vi "maszyna stanowa 1.vi"(6 "Niewykonane eventy in":T1[](array[typedef]), 8 "Ile godzin":i32=1, 9 "Liczba klientów na godzinę":i32=100, 10 "Sklep in":T2={"kasy"=2, "wolne"=2, "zarobek"=0, "liczba klientów"=0, "czas w kolejce"=0}, 11 "queue in":refnum<queue>) -> (0 "Straceni klienci":i32, 1 "Niewykonane eventy out":T1[](array[typedef]), 2 "Sklep out":T2={"kasy"=2, "wolne"=2, "zarobek"=0, "liczba klientów"=0, "czas w kolejce"=0}, 3 "queue out":refnum<queue>)   [LabVIEW 2013]
uses:
  event.ctl
  sklep.ctl
panel:
  out "liczba klientów":i32
  out "zarobek":i32
  out "średni czas w kolejce":dbl
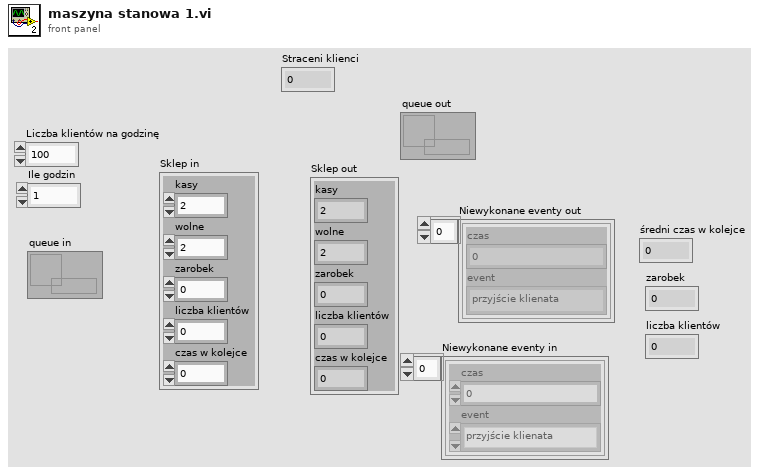
[diagram p1: front panel]
types:
  T1 = typedef "event.ctl" = cluster{"czas":u32, "event":enum16{"przyjście klienata", "zwolnienie kasy", "oczekiwanie na klienta", "nowy event"}}
  T2 = typedef "sklep.ctl" = cluster{"kasy":i32, "wolne":i32, "zarobek":i32, "liczba klientów":i32, "czas w kolejce":u64}
  T3 = enum16{"przyjście klienata", "zwolnienie kasy", "oczekiwanie na klienta", "nowy event"}
  T4 = cluster{dbl, "event":enum16{"przyjście klienata", "zwolnienie kasy", "oczekiwanie na klienta", "nowy event"}}
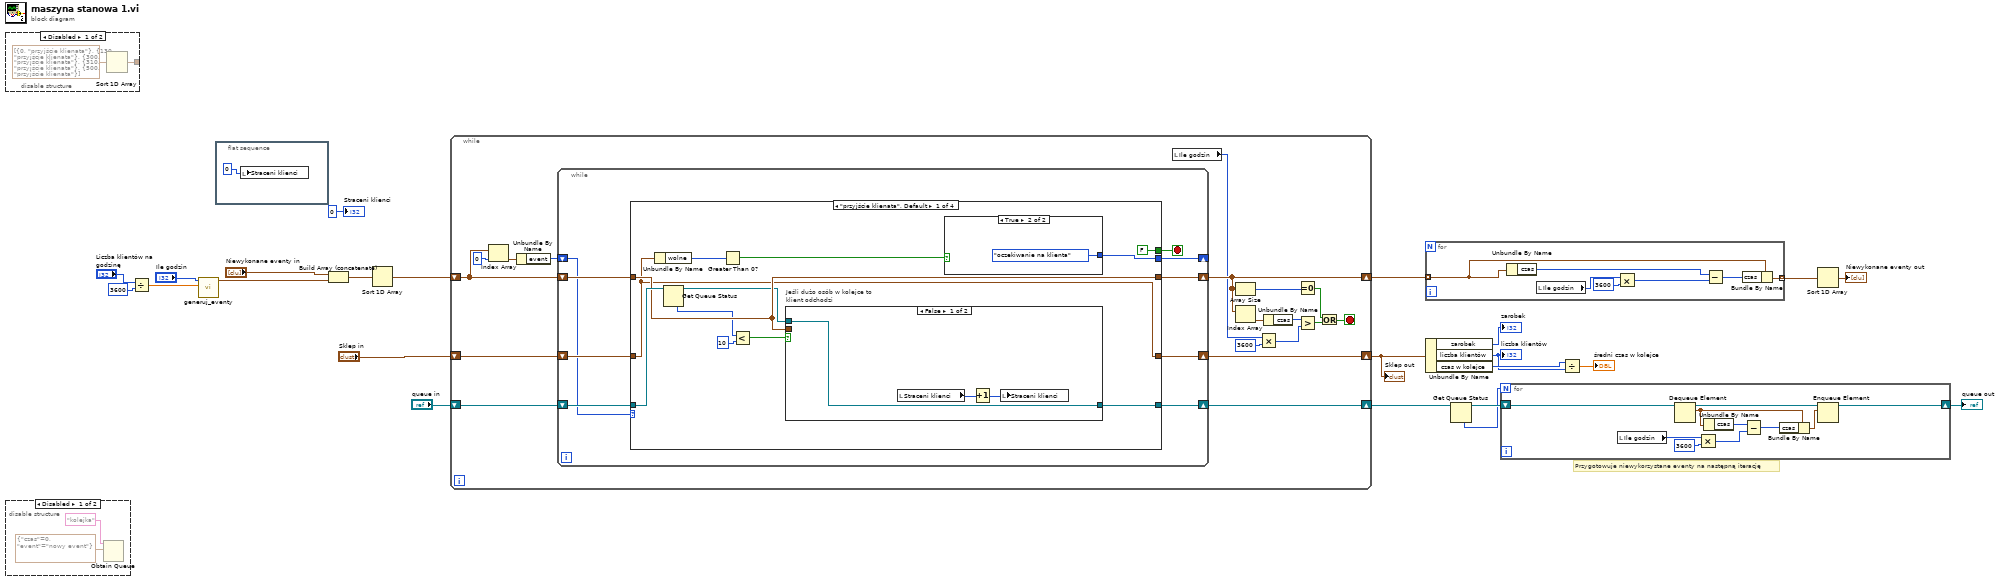
[diagram p0: block diagram]
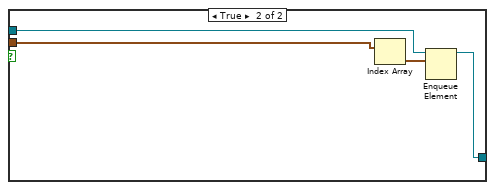
[diagram p4: hidden frame]
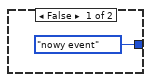
[diagram p5: hidden frame]
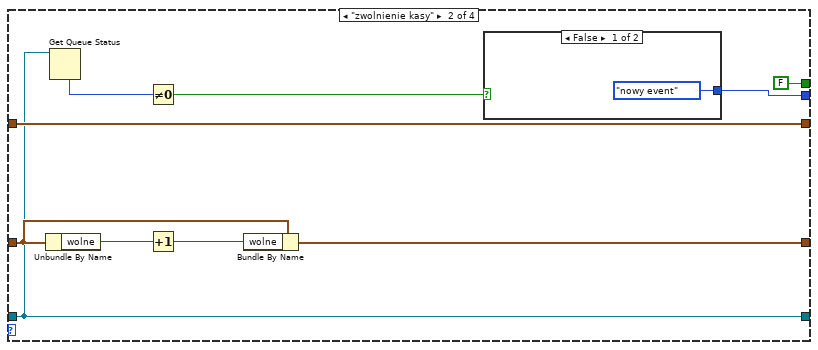
[diagram p6: hidden frame]
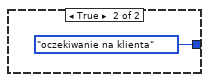
[diagram p7: hidden frame]
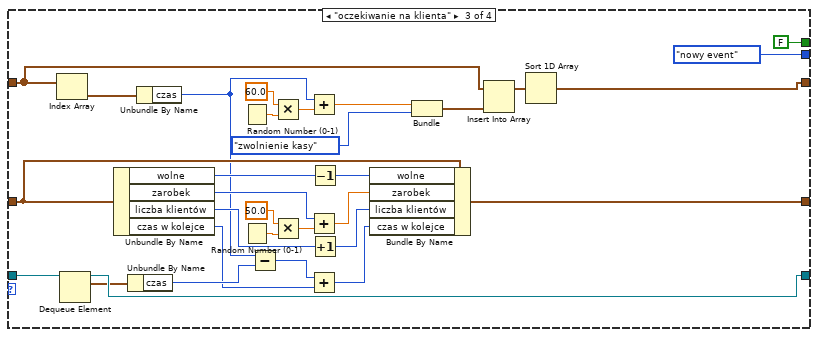
[diagram p8: hidden frame]
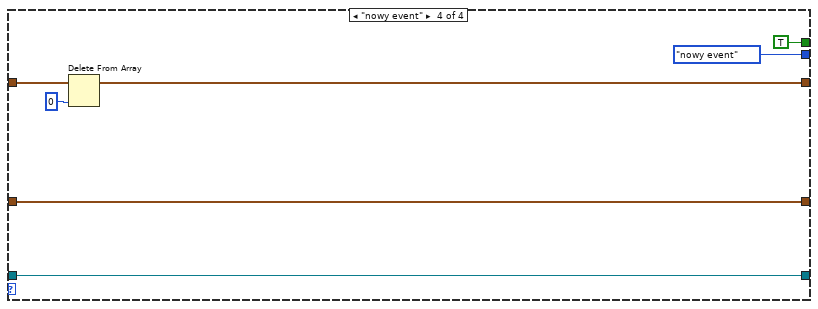
[diagram p9: hidden frame]
diagram:
  # "Przygotowuje niewykorzystane eventy na następną iterację"
  n1 = disable-structure shown="Disabled" {
    disable-tunnel: [w24 _] -> _
    frame Disabled {
      n2 = Sort 1D Array(array=T1[] [{"czas"=0, "event"=enum."przyjście klienata"}, {"czas"=130, "event"=enum."przyjście klienata"}, {"czas"=300, "event"=enum."przyjście klienata"}, {"czas"=310, "event"=enum."przyjście klienata"}, {"czas"=500, "event"=enum."przyjście klienata"}]) -> (sorted array=w24:T1[])
    }
    frame Enabled {
    }
  }
  n3 = disable-structure shown="Disabled" {
    frame Disabled {
      n4 = Obtain Queue(name (unnamed)="kolejka", element data type=T1 {"czas"=0, "event"=enum."nowy event"} ("Cluster")) -> ()  [unwired: 3 in, 3 out]
    }
    frame Enabled {
    }
  }
  n5 = Divide(x="Liczba klientów na godzinę", y=3600) -> (x/y=w20:dbl)
  n6 = call "generuj_eventy.vi"("lambda"=w20, "Godziny"="Ile godzin") -> ("Array"=w15:T1[])  [unwired: 9 in]
  n7 = flat-sequence {
    frame #0 {
      n8 = local write "Straceni klienci"(0) -> ()
    }
  }
  n9 = Build Array (concatenate)("Niewykonane eventy in", w15) -> (w14:T1[])
  n10 = Sort 1D Array(array=w14) -> (sorted array=w13:T1[])
  n11 = while {
    shift-right: [w39] -> w8
    shift-left: "Sklep in" -> [w43]
    shift-right: [w40] -> w6
    shift-left: "queue in" -> [w44]
    shift-right: [w37] -> w18
    shift-left: w13 -> [w45]
    stop <- w32 stop-if-true
    n12 = Index Array(array=w45, index=0) -> (element=w42:T1)
    n13 = Unbundle By Name(w42) -> ("event"=w41:T3)
    n14 = while {
      shift-right: [w51] -> _
      shift-left: w41 -> [w52]
      shift-right: [w49] -> w39
      shift-left: w43 -> [w53]
      shift-right: [w50] -> w40
      shift-left: w44 -> [w54]
      shift-right: [w48] -> w37
      shift-left: w45 -> [w55]
      stop <- w47 stop-if-true
      n15 = case shown="\"przyjście klienata\", Default" w52 {
        tunnel: w55 -> [w62 w79 w99 w126]
        tunnel: w54 -> [w67 w77 w113 w122]
        tunnel: w53 -> [w61 w85 w106 w121]
        tunnel: [w64 w80 T3."nowy event" ("event") T3."nowy event" ("event")] -> w51
        tunnel: [w63 w77 w112 w122] -> w50
        tunnel: [w61 w83 w101 w121] -> w49
        tunnel: [w62 w79 w90 w124] -> w48
        tunnel: [FALSE FALSE FALSE TRUE] -> w47
        frame "przyjście klienata", Default {
          n16 = Unbundle By Name(w61) -> ("wolne"=w66:i32)
          n17 = Get Queue Status(queue=w67) -> (queue out=w59:refnum<queue>, # elements in queue=w58:i32)  [unwired: 2 in, 6 out]
          n18 = Greater Than 0?(x=w66) -> (x > 0?=w65:bool)
          n19 = Less?(x=w58, y=10) -> (x < y?=w56:bool)
          n20 = case "Jeśli dużo osób w kolejce to \nklient odchodzi" shown="False" w56 {
            tunnel: w59 -> [w70 w74]
            tunnel: [w70 w72] -> w63
            tunnel: w62 -> [_ w71]
            frame False {
              n21 = local read "Straceni klienci"() -> (w69:i32)
              n22 = Increment(x=w69) -> (x+1=w68:i32)
              n23 = local write "Straceni klienci"(w68) -> ()
            }
            frame True {
              n24 = Index Array(array=w71) -> (element=w73:T1)  [unwired: 1 in]
              n25 = Enqueue Element(queue=w74, element=w73) -> (queue out=w72:refnum<queue>)  [unwired: 2 in, 2 out]
            }
          }
          n26 = case shown="True" w65 {
            tunnel: [T3."nowy event" ("event") T3."oczekiwanie na klienta" ("event")] -> w64
            frame False {
            }
            frame True {
            }
          }
        }
        frame "zwolnienie kasy" {
          n27 = Unbundle By Name(w85) -> ("wolne"=w86:i32)
          n28 = Get Queue Status(queue=w77) -> (# elements in queue=w82:i32)  [unwired: 2 in, 7 out]
          n29 = Not Equal To 0?(x=w82) -> (x != 0?=w81:bool)
          n30 = Increment(x=w86) -> (x+1=w84:i32)
          n31 = Bundle By Name(cluster=w85, "wolne"=w84) -> (w83:T2)
          n32 = case shown="False" w81 {
            tunnel: [T3."nowy event" ("event") T3."oczekiwanie na klienta" ("event")] -> w80
            frame False {
            }
            frame True {
            }
          }
        }
        frame "oczekiwanie na klienta" {
          n33 = Index Array(array=w99) -> (element=w110:T1)  [unwired: 1 in]
          n34 = Dequeue Element(queue=w113) -> (queue out=w112:refnum<queue>, element=w111:T1)  [unwired: 2 in, 2 out]
          n35 = Unbundle By Name(w106) -> ("wolne"=w119:i32, "zarobek"=w117:i32, "liczba klientów"=w114:i32, "czas w kolejce"=w108:u64)
          n36 = Unbundle By Name(w111) -> ("czas"=w109:u32)
          n37 = Unbundle By Name(w110) -> ("czas"=w98:u32)
          n38 = Random Number (0-1)() -> (number: 0 to 1=w95:dbl)
          n39 = Random Number (0-1)() -> (number: 0 to 1=w116:dbl)
          n40 = Subtract(x=w98, y=w109) -> (x-y=w107:u32)
          n41 = Multiply(x=60.0, y=w95) -> (x*y=w97:dbl)
          n42 = Multiply(x=50.0, y=w116) -> (x*y=w118:dbl)
          n43 = Add(x=w98, y=w97) -> (x+y=w94:dbl)
          n44 = Add(x=w117, y=w118) -> (x+y=w104:dbl)
          n45 = Add(x=w107, y=w108) -> (x+y=w102:u64)
          n46 = Decrement(x=w119) -> (x-1=w105:i32)
          n47 = Increment(x=w114) -> (x+1=w103:i32)
          n48 = Bundle By Name(cluster=w106, "wolne"=w105, "zarobek"=w104, "liczba klientów"=w103, "czas w kolejce"=w102) -> (w101:T2)
          n49 = Bundle(w94, "event"=T3."zwolnienie kasy") -> (w92:T4)  [unwired: 1 in]
          n50 = Insert Into Array(array=w99, new element=w92) -> (w91:T1[])  [unwired: 1 in]
          n51 = Sort 1D Array(array=w91) -> (sorted array=w90:T1[])
        }
        frame "nowy event" {
          n52 = Delete From Array(array=w126, index=0) -> (array with subset deleted=w124:T1[])  [unwired: 1 in, 1 out]
        }
      }
    }
    n53 = local read "Ile godzin"() -> (w31:i32)
    n54 = Array Size(array=w37) -> (size(s)=w38:i32)
    n55 = Index Array(array=w37) -> (element=w36:T1)  [unwired: 1 in]
    n56 = Multiply(x=w31, y=3600) -> (x*y=w29:i32)
    n57 = Unbundle By Name(w36) -> ("czas"=w35:u32)
    n58 = Equal To 0?(x=w38) -> (x = 0?=w33:bool)
    n59 = Greater?(x=w35, y=w29) -> (0:w34:bool)
    n60 = Or(x=w33, y=w34) -> (x .or. y?=w32:bool)
  }
  "Sklep out" <- w8
  n61 = for {
    tunnel: w18 -> [w131] mode=indexing
    tunnel: [w127] -> w17 mode=indexing
    n62 = Unbundle By Name(w131) -> ("czas"=w130:u32)
    n63 = local read "Ile godzin"() -> (w133:i32)
    n64 = Multiply(x=w133, y=3600) -> (x*y=w129:i32)
    n65 = Subtract(x=w130, y=w129) -> (x-y=w128:u32)
    n66 = Bundle By Name(cluster=w131, "czas"=w128) -> (w127:T1)
  }
  n67 = Unbundle By Name(w8) -> ("zarobek"=→"zarobek":i32, "liczba klientów"=w11:i32, "czas w kolejce"=w12:u64)
  "liczba klientów" <- w11
  n68 = Get Queue Status(queue=w6) -> (queue out=w5:refnum<queue>, # elements in queue=w4:i32)  [unwired: 2 in, 6 out]
  n69 = for {
    N: w4 -> [_]
    shift-right: [w137] -> w3
    shift-left: w5 -> [w141]
    n70 = local read "Ile godzin"() -> (w142:i32)
    n71 = Dequeue Element(queue=w141) -> (queue out=w140:refnum<queue>, element=w139:T1)  [unwired: 2 in, 2 out]
    n72 = Multiply(x=w142, y=3600) -> (x*y=w134:i32)
    n73 = Unbundle By Name(w139) -> ("czas"=w135:u32)
    n74 = Subtract(x=w135, y=w134) -> (x-y=w136:u32)
    n75 = Bundle By Name(cluster=w139, "czas"=w136) -> (w138:T1)
    n76 = Enqueue Element(queue=w140, element=w138) -> (queue out=w137:refnum<queue>)  [unwired: 2 in, 2 out]
  }
  "queue out" <- w3
  n77 = Divide(x=w12, y=w11) -> (x/y=→"średni czas w kolejce":dbl)
  n78 = Sort 1D Array(array=w17) -> (sorted array=→"Niewykonane eventy out":T1[])
  "Straceni klienci" <- 0
